vi "LitePoint_TRXConfiguration.vi"(8 "error in (no error)":errorcluster, 10 "TRXmode":u16(ring) items=["Tx", "Rx"], 11 "VISA resource name":refnum<visa-resource-name>) -> (0 "error out":errorcluster, 3 "VISA resource name out":refnum<visa-resource-name>)   [LabVIEW 2020, in "LitePoints.lvlib"]
uses:
  LitePoints.lvlib
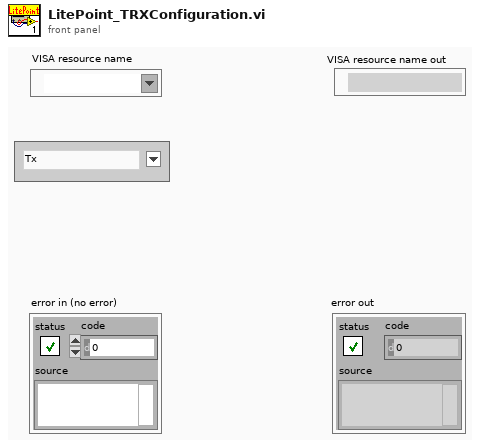
[diagram p1: front panel]
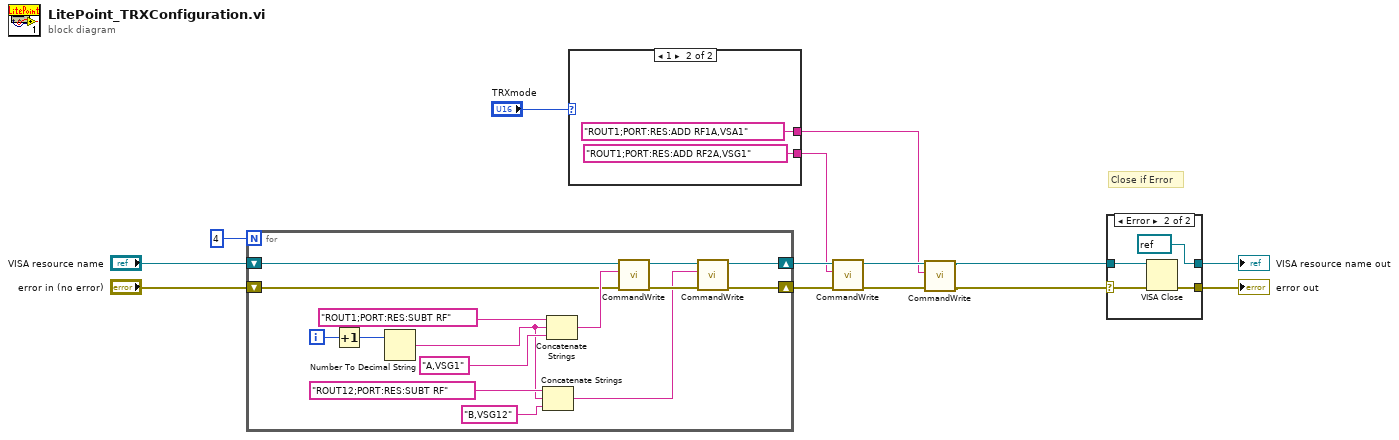
[diagram p0: block diagram]
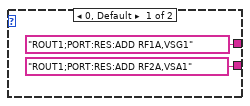
[diagram p2: hidden frame]
diagram:
  # "Close if Error"
  n1 = for {
    N: 4 -> [_]
    shift-right: [w16] -> w8
    shift-left: "VISA resource name" -> [w17]
    shift-right: [w15] -> w9
    shift-left: "error in (no error)" -> [w18]
    i -> [w27]
    n2 = Increment(x=w27) -> (x+1=w28:i32)
    n3 = Number To Decimal String(number=w28) -> (decimal integer string=w24:string)  [unwired: 1 in]
    n4 = Concatenate Strings("ROUT12;PORT:RES:SUBT RF", w24, "B,VSG12") -> (w19:string)
    n5 = Concatenate Strings("ROUT1;PORT:RES:SUBT RF", w24, "A,VSG1") -> (w22:string)
    n6 = call "CommandWrite.vi"("error in (no error)"=w18, "Write Buffer"=w22, "VISA resource name"=w17) -> ("error out"=w21:errorcluster, "VISA resource name out"=w20:refnum<visa-resource-name>)  [unwired: 7 in]
    n7 = call "CommandWrite.vi"("error in (no error)"=w21, "Write Buffer"=w19, "VISA resource name"=w20) -> ("error out"=w15:errorcluster, "VISA resource name out"=w16:refnum<visa-resource-name>)  [unwired: 7 in]
  }
  n8 = case shown="1" "TRXmode" {
    tunnel: ["ROUT1;PORT:RES:ADD RF2A,VSA1" "ROUT1;PORT:RES:ADD RF2A,VSG1"] -> w2
    tunnel: ["ROUT1;PORT:RES:ADD RF1A,VSG1" "ROUT1;PORT:RES:ADD RF1A,VSA1"] -> w1
    frame 0, Default {
    }
    frame 1 {
    }
  }
  n9 = call "CommandWrite.vi"("error in (no error)"=w9, "Write Buffer"=w2, "VISA resource name"=w8) -> ("error out"=w4:errorcluster, "VISA resource name out"=w5:refnum<visa-resource-name>)  [unwired: 7 in]
  n10 = call "CommandWrite.vi"("error in (no error)"=w4, "Write Buffer"=w1, "VISA resource name"=w5) -> ("error out"=w6:errorcluster, "VISA resource name out"=w7:refnum<visa-resource-name>)  [unwired: 7 in]
  n11 = case shown="Error" w6 {
    selector: w6 -> [w34 w37]
    tunnel: w7 -> [w35 w38]
    tunnel: [w35 refnum<visa-resource-name> refnum ("VISA resource name out")] -> w14
    tunnel: [w34 w36] -> w13
    frame No Error {
    }
    frame Error {
      n12 = VISA Close(VISA resource name=w38, error in (no error)=w37) -> (error out=w36:errorcluster)
    }
  }
  "VISA resource name out" <- w14
  "error out" <- w13
